vi "Init Msg Input.vi"(6 "Teller":T1 {"Absolute Time" format="%<%x %.3X>T"}) -> (3 "Start Msg Input out":refnum<class "Start Msg Input.lvclass">)   [LabVIEW 2020, in "jettl.lvlib" / "Start jettl Msg.lvlib" / "Start Msg Input.lvlib" / "Start Msg Input.lvclass"]
doc: "jettl 6.14.1.98\nNathan Davis - Nathan Davis\nCopyright (c) 2026, Nathan Davis\nMIT"
uses:
  Start Msg Input.lvclass
  Teller Metadata/Teller Metadata.lvclass
  Start Msg Input.lvclass/Start Msg Input.ctl
  Relation.ctl
  jettl.lvlib
  Teller.ctl
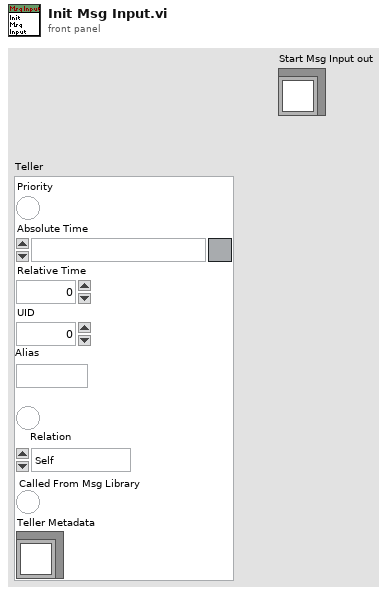
[diagram p1: front panel]
types:
  T1 = typedef "jettl.lvlib/Teller.ctl" = cluster{"Priority":bool, "Absolute Time":timestamp, "Relative Time":dbl, "UID":i32, "Alias":string, "Valid Relation":bool, "Relation":T2, "Called From Msg Library":bool, "Teller Metadata":refnum<class "Teller Metadata.lvclass">}
  T2 = typedef "jettl.lvlib/Relation.ctl" = enum16{"Self", "Parent", "Child"}
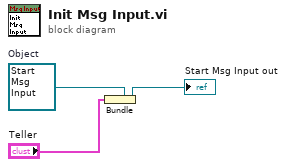
[diagram p0: block diagram]
diagram:
  w3 = refnum<class "Start Msg Input.lvclass"> refnum  # Object
  n1 = Bundle "Bundle"(cluster=w3, "Teller") -> (→"Start Msg Input out":refnum<class "Start Msg Input.lvclass">)
